vi "Testing.vi"() -> ()   [LabVIEW 2009]
panel:
  in  "N_PolCoeff":i32=1
  in  "Polynomial Coefficients":sgl[](array[numeric])=[1.0, 0.0, 0.0, 0.0, 0.0, 0.0, 0.0, 0.0, 0.0, 0.0, 0.0, 0.0, 0.0, 0.0, 0.0, 0.0, 0.0, 0.0, 0.0, 0.0, 0.0, 0.0, 0.0, 0.0, 0.0, 0.0, 0.0, 0.0, 0.0, 0.0, 0.0, 0.0, 0.0, 0.0, 0.0, 0.0, 0.0, 0.0, 0.0, 0.0, 0.0, 0.0, 0.0, 0.0, 0.0, 0.0, 0.0, 0.0, 0.0, 0.0, 0.0, 0.0, 0.0, 0.0, 0.0, 0.0, 0.0, 0.0, 0.0, 0.0, 0.0, 0.0, 0.0, 0.0, 0.0, 0.0, 0.0, 0.0, 0.0, 0.0, 0.0, 0.0, 0.0, 0.0, 0.0, 0.0, 0.0, 0.0, 0.0, 0.0, 0.0, 0.0, 0.0, 0.0, 0.0, 0.0, 0.0, 0.0, 0.0, 0.0, 0.0, 0.0, 0.0, 0.0, 0.0, 0.0, 0.0, 0.0, 0.0, 0.0, 0.0, 0.0, 0.0, 0.0, 0.0, 0.0, 0.0, 0.0, 0.0, 0.0, 0.0, 0.0, 0.0, 0.0, 0.0, 0.0, 0.0, 0.0, 0.0, 0.0]
  in  "Aberration Correction":sgl[](array[numeric])=array[262144 elements]
  out "error out":errorcluster
  out "CUDA return 2":i32
  out "CUDA Return 1":i32
  in  "Use polynomial LUT":bool
  in  "Aberration Correction On":bool
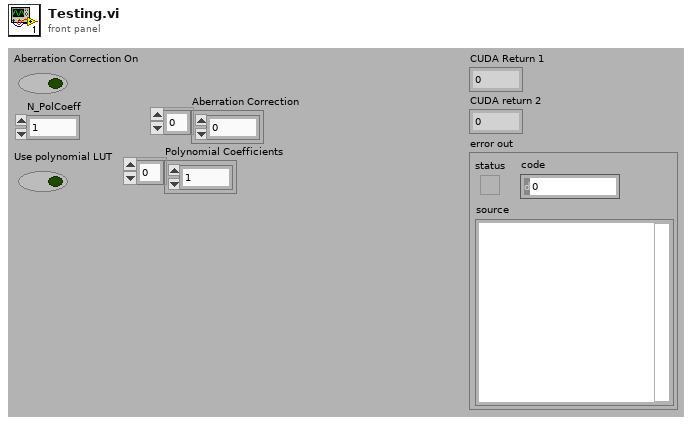
[diagram p1: front panel]
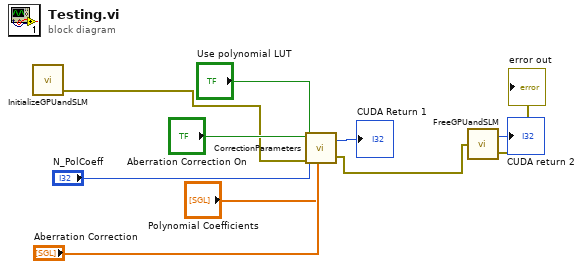
[diagram p0: block diagram]
diagram:
  n1 = call "InitializeGPUandSLM.vi"() -> ("CUDA/SLM error"=w6:errorcluster)  [unwired: 4 in, 1 out]
  n2 = call "CorrectionParameters.vi"("Polynomial Coefficients"="Polynomial Coefficients", "Aberration Correction"="Aberration Correction", "error in"=w6, "N_PolCoeff"="N_PolCoeff", "Use polynomial LUT"="Use polynomial LUT", "Aberration Correction On"="Aberration Correction On") -> ("error out"=w7:errorcluster, "CUDA Return"=→"CUDA Return 1":i32)
  n3 = call "FreeGPUandSLM.vi"("error in"=w7) -> ("CUDA return"=→"CUDA return 2":i32, "error out"=→"error out":errorcluster)
